vi "Serial Channel IO.vi"(0 "arm":bool, 1 "reset":bool, 2 "common resources":T15={"sync pulse resources"={"sync pulse destination terminal"="", "sync100"="", "sync pulse source terminal"="", "imported sync pulse register"="", "generate sync pulse handshake"="", "enable sync pulse register"="", "sync pulse clock"=""}, "serial channel resources"={"sc 0"={"completed frames register"=""}, "sc 1"={"completed frames register"=""}, "sc 2"={"completed frames register"=""}, "sc 3"={"completed frames register"=""}, "sc 4"={"completed frames register"=""}, "sc 5"={"completed frames register"=""}, "sc 6"={"completed frames register"=""}, "sc 7"={"completed frames register"=""}}, "dram manager 0"={"DRAM class"=refnum, "process clock"="", "registers"={"configuration"={"write time slice"="", "request time slice"="", "DRAM arbiter config"="", "partition config"=""}, "reset"={"handshake"={"start.go"="", "start.go rcvd"="", "done.go"="", "done.go rcvd"=""}, "process"={"in"="", "out"=""}, "write"={"in"="", "out 0"="", "out 1"="", "out 2"="", "out 3"=""}, "read"={"in"="", "out 0"="", "out 1"="", "out 2"="", "out 3"=""}}, "status"={"partition full"=""}}, "FIFOs"={"write data"={"FIFO 0"="", "FIFO 1"="", "FIFO 2"="", "FIFO 3"=""}, "request metadata"={"FIFO"=""}, "read data VOQ"={"FIFO 0"="", "FIFO 1"="", "FIFO 2"="", "FIFO 3"=""}, "read data"={"FIFO 0"="", "FIFO 1"="", "FIFO 2"="", "FIFO 3"=""}}, "num active streams"=0.0, "max open read requests"=256}, "dram manager 1"={"DRAM class"=refnum, "process clock"="", "registers"={"configuration"={"write time slice"="", "request time slice"="", "DRAM arbiter config"="", "partition config"=""}, "reset"={"handshake"={"start.go"="", "start.go rcvd"="", "done.go"="", "done.go rcvd"=""}, "process"={"in"="", "out"=""}, "write"={"in"="", "out 0"="", "out 1"="", "out 2"="", "out 3"=""}, "read"={"in"="", "out 0"="", "out 1"="", "out 2"="", "out 3"=""}}, "status"={"partition full"=""}}, "FIFOs"={"write data"={"FIFO 0"="", "FIFO 1"="", "FIFO 2"="", "FIFO 3"=""}, "request metadata"={"FIFO"=""}, "read data VOQ"={"FIFO 0"="", "FIFO 1"="", "FIFO 2"="", "FIFO 3"=""}, "read data"={"FIFO 0"="", "FIFO 1"="", "FIFO 2"="", "FIFO 3"=""}}, "num active streams"=0.0, "max open read requests"=256}}, 5 "stop":bool, 7 "timestamp counter value":T26, 9 "channel configs":T11[](array[typedef]) {"channel acq config"."first packet data type select mask" format="%.0x"; "channel acq config"."last packet data type select mask" format="%.0x"}, 11 "dram partition configs":T14[](array[typedef])=[{"first address"=0, "last address"=0}, {"first address"=0, "last address"=0}, {"first address"=0, "last address"=0}, {"first address"=0, "last address"=0}, {"first address"=0, "last address"=0}, {"first address"=0, "last address"=0}, {"first address"=0, "last address"=0}, {"first address"=0, "last address"=0}], 12 "ready for output":bool[](array[boolean])=[TRUE, TRUE, TRUE, TRUE, TRUE, TRUE, TRUE, TRUE]) -> (3 "acquisition error":bool, 4 "tagged llp packets cluster":T1, 6 "end of data":bool[](array[boolean]), 8 "serial input channel status":T27[](array[typedef])=[{"acq state"=enum."Idle", "stop timed out"=FALSE, "bad packet header"=FALSE, "bad packet payload"=FALSE, "bad packet size"=FALSE, "dram status"={"bytes written"=0, "bytes read"=0, "overflow"=FALSE, "partition full"=FALSE, "last byte flushed"=FALSE}}, {"acq state"=enum."Idle", "stop timed out"=FALSE, "bad packet header"=FALSE, "bad packet payload"=FALSE, "bad packet size"=FALSE, "dram status"={"bytes written"=0, "bytes read"=0, "overflow"=FALSE, "partition full"=FALSE, "last byte flushed"=FALSE}}, {"acq state"=enum."Idle", "stop timed out"=FALSE, "bad packet header"=FALSE, "bad packet payload"=FALSE, "bad packet size"=FALSE, "dram status"={"bytes written"=0, "bytes read"=0, "overflow"=FALSE, "partition full"=FALSE, "last byte flushed"=FALSE}}, {"acq state"=enum."Idle", "stop timed out"=FALSE, "bad packet header"=FALSE, "bad packet payload"=FALSE, "bad packet size"=FALSE, "dram status"={"bytes written"=0, "bytes read"=0, "overflow"=FALSE, "partition full"=FALSE, "last byte flushed"=FALSE}}, {"acq state"=enum."Idle", "stop timed out"=FALSE, "bad packet header"=FALSE, "bad packet payload"=FALSE, "bad packet size"=FALSE, "dram status"={"bytes written"=0, "bytes read"=0, "overflow"=FALSE, "partition full"=FALSE, "last byte flushed"=FALSE}}, {"acq state"=enum."Idle", "stop timed out"=FALSE, "bad packet header"=FALSE, "bad packet payload"=FALSE, "bad packet size"=FALSE, "dram status"={"bytes written"=0, "bytes read"=0, "overflow"=FALSE, "partition full"=FALSE, "last byte flushed"=FALSE}}, {"acq state"=enum."Idle", "stop timed out"=FALSE, "bad packet header"=FALSE, "bad packet payload"=FALSE, "bad packet size"=FALSE, "dram status"={"bytes written"=0, "bytes read"=0, "overflow"=FALSE, "partition full"=FALSE, "last byte flushed"=FALSE}}, {"acq state"=enum."Idle", "stop timed out"=FALSE, "bad packet header"=FALSE, "bad packet payload"=FALSE, "bad packet size"=FALSE, "dram status"={"bytes written"=0, "bytes read"=0, "overflow"=FALSE, "partition full"=FALSE, "last byte flushed"=FALSE}}], 10 "tagged llp packet valid":bool[](array[boolean]), 14 "ready for arm":bool, 15 "i2c monitor array":T13[](array[typedef]) {"monitor word" format="%.0x"})   [LabVIEW 2020, in "GettingStarted_Acq_Tap_148X_FPGA.lvlib"]
uses:
  GettingStarted_Acq_Tap_148X_FPGA.lvlib
  Types/Serial Input Channel Status.ctl
  <instrlib>/FlexRIO/CSI-2/v2/FPGA/Types/Channel-Based Acquisition Engine State.ctl
  Common/Types/DRAM Status.ctl
  <instrlib>/FlexRIO/CSI-2/v2/FPGA/Types/Timestamp Counter Value.ctl
  Common/Types/Common Resources.ctl
  <instrlib>/_niInstr/Memory/v1/FPGA/DRAM/niInstr Memory DRAM v1 FPGA.lvclass
  <instrlib>/FlexRIO/CSI-2/v2/FPGA/Types/Sync Pulse Resources.ctl
  Common/Types/Serial Channel Resources.ctl
  Common/Types/Single Serial Channel Resources.ctl
  <instrlib>/FlexRIO/CSI-2/v2/FPGA/DRAM Manager/Private/DRAM Manager.ctl
  <instrlib>/FlexRIO/CSI-2/v2/FPGA/DRAM Manager/Private/Common/DRAM Manager Registers.ctl
  <instrlib>/FlexRIO/CSI-2/v2/FPGA/DRAM Manager/Private/Common/Handshake Registers.ctl
  <instrlib>/FlexRIO/CSI-2/v2/FPGA/DRAM Manager/Private/Common/DRAM Manager FIFOs.ctl
  <instrlib>/FlexRIO/CSI-2/v2/FPGA/DRAM Manager/Private/Common/Write Data FIFO Ref.ctl
  <instrlib>/FlexRIO/CSI-2/v2/FPGA/DRAM Manager/Private/Common/Read Request Metadata FIFO Ref.ctl
  <instrlib>/FlexRIO/CSI-2/v2/FPGA/DRAM Manager/Private/Common/Read Data FIFO Ref.ctl
  <instrlib>/FlexRIO/CSI-2/v2/FPGA/DRAM Manager/Public/Partition Range.ctl
  <instrlib>/FlexRIO/API/FPGA/v1/IO/NI148x/i2c monitor.ctl
  Types/Serial Input Channel Datapath Configuration.ctl
  <instrlib>/FlexRIO/CSI-2/v2/FPGA/Types/Channel-Based Acquistion Engine Configuration.ctl
  Common/Types/Tagged LLP Packets Cluster.ctl
  <instrlib>/FlexRIO/CSI-2/v2/FPGA/Types/Tagged LLP Packet.ctl
  <instrlib>/FlexRIO/CSI-2/v2/FPGA/Types/FPGA LLP Packet Tag.ctl
  <instrlib>/FlexRIO/CSI-2/v2/FPGA/Types/FPGA LLP Packet Timestamp.ctl
  <instrlib>/FlexRIO/CSI-2/v2/FPGA/Types/Timestamp ID.ctl
  <instrlib>/FlexRIO/CSI-2/v2/FPGA/Types/FPGA LLP Packet Size.ctl
  <instrlib>/FlexRIO/CSI-2/v2/FPGA/Types/LLP Packet.ctl
  <instrlib>/FlexRIO/CSI-2/v2/FPGA/Types/LLP Packet Header.ctl
  <instrlib>/FlexRIO/CSI-2/v2/FPGA/Types/LLP Packet Payload.ctl
  <instrlib>/FlexRIO/CSI-2/v2/FPGA/Types/LLP Packet Footer.ctl
  <instrlib>/_niInstr/Basic Elements/v1/FPGA/niInstr Basic Elements v1 FPGA.lvlib
  Common/GettingStarted_Common_148X_FPGA.lvlib
  <instrlib>/FlexRIO/CSI-2/v2/FPGA/NI CSI-2 API FPGA v2.lvlib
  <instrlib>/FlexRIO/CSI-2/v2/FPGA/DRAM Manager/DRAM Manager v2.lvlib
  <instrlib>/FlexRIO/API/FPGA/v1/IO/NI148x/FlexRIO 148x FPGA v1.lvlib
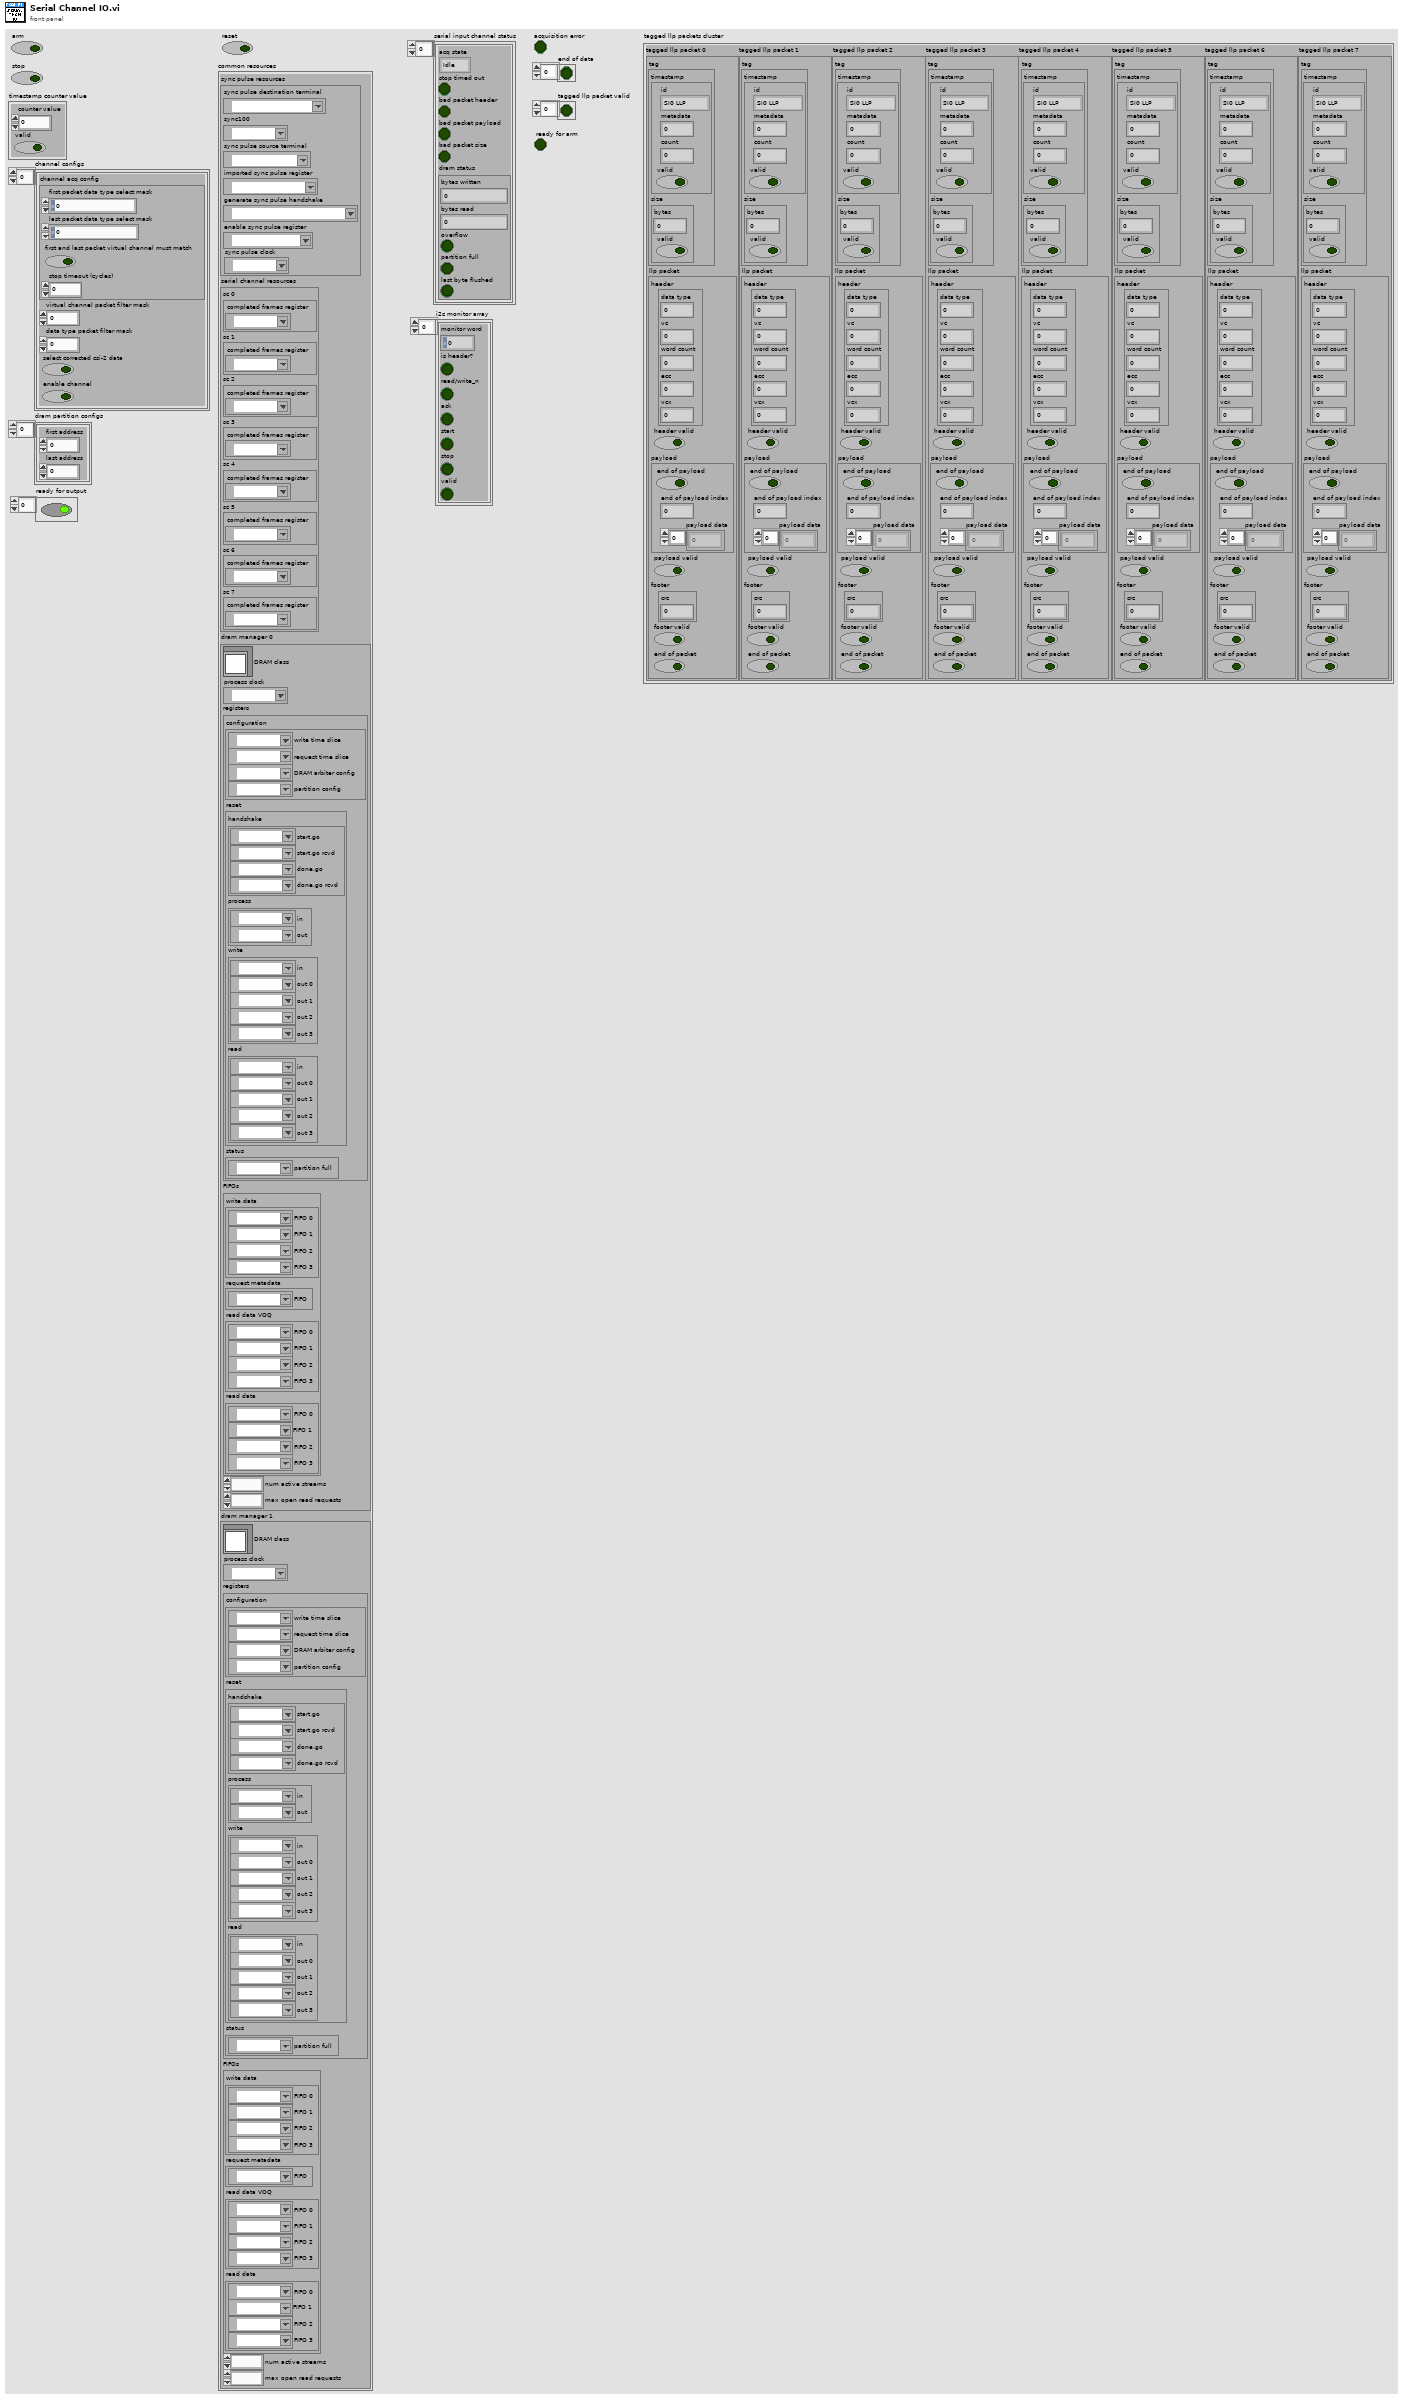
[diagram p1: front panel]
types:
  T1 = typedef "GettingStarted_Common_148X_FPGA.lvlib/Tagged LLP Packets Cluster.ctl" = cluster{"tagged llp packet 0":T2, "tagged llp packet 1":T2, "tagged llp packet 2":T2, "tagged llp packet 3":T2, "tagged llp packet 4":T2, "tagged llp packet 5":T2, "tagged llp packet 6":T2, "tagged llp packet 7":T2}
  T2 = typedef "NI CSI-2 API FPGA v2.lvlib/Tagged LLP Packet.ctl" = cluster{"tag":T3, "llp packet":T7}
  T3 = typedef "NI CSI-2 API FPGA v2.lvlib/FPGA LLP Packet Tag.ctl" = cluster{"timestamp":T4, "size":T6}
  T4 = typedef "NI CSI-2 API FPGA v2.lvlib/FPGA LLP Packet Timestamp.ctl" = cluster{"valid":bool, "count":fxp<+,50,50>, "id":T5, "metadata":u8}
  T5 = typedef "NI CSI-2 API FPGA v2.lvlib/Timestamp ID.ctl" = enum8{"SI0 LLP", "SI1 LLP", "SI2 LLP", "SI3 LLP", "SI4 LLP", "SI5 LLP", "SI6 LLP", "SI7 LLP", "SO0 LLP", "SO1 LLP", "SO2 LLP", "SO3 LLP", "SO4 LLP", "SO5 LLP", "SO6 LLP", "SO7 LLP", "Ser0 GPIO Bank", "Ser1 GPIO Bank", "Ser2 GPIO Bank", "Ser3 GPIO Bank", "Ser4 GPIO Bank", "Ser5 GPIO Bank", "Ser6 GPIO Bank", "Ser7 GPIO Bank", "Des0 GPIO Bank", "Des1 GPIO Bank", "Des2 GPIO Bank", "Des3 GPIO Bank", "Des4 GPIO Bank", "Des5 GPIO Bank", "Des6 GPIO Bank", "Des7 GPIO Bank", "User0", "User1", "User2", "User3", "User4", "User5", "User6", "User7", "User8", "User9", "User10", "User11", "User12", "User13", "User14", "User15", "User16", "User17", "User18", "User19", "User20", "User21", "User22", "User23", "User24", "User25", "User26", "User27", "User28", "User29", "User30", "User31"}
  T6 = typedef "NI CSI-2 API FPGA v2.lvlib/FPGA LLP Packet Size.ctl" = cluster{"bytes":fxp<+,17,17>, "valid":bool}
  T7 = typedef "NI CSI-2 API FPGA v2.lvlib/LLP Packet.ctl" = cluster{"header":T8, "header valid":bool, "payload":T9, "payload valid":bool, "footer":T10, "footer valid":bool, "end of packet":bool}
  T8 = typedef "NI CSI-2 API FPGA v2.lvlib/LLP Packet Header.ctl" = cluster{"word count":u16, "ecc":fxp<+,6,6>, "vcx":fxp<+,2,2>, "data type":fxp<+,6,6>, "vc":fxp<+,2,2>}
  T9 = typedef "NI CSI-2 API FPGA v2.lvlib/LLP Packet Payload.ctl" = cluster{"end of payload":bool, "end of payload index":fxp<+,3,3>, "payload data":u8[]}
  T10 = typedef "NI CSI-2 API FPGA v2.lvlib/LLP Packet Footer.ctl" = cluster{"crc":u16}
  T11 = typedef "GettingStarted_Acq_Tap_148X_FPGA.lvlib/Serial Input Channel Datapath Configuration.ctl" = cluster{"channel acq config":T12, "virtual channel packet filter mask":u16, "data type packet filter mask":u64, "select corrected csi-2 data":bool, "enable channel":bool}
  T12 = typedef "NI CSI-2 API FPGA v2.lvlib/Channel-Based Acquistion Engine Configuration.ctl" = cluster{"stop timeout (cycles)":u32, "first packet data type select mask":u64, "last packet data type select mask":u64, "first and last packet virtual channel must match":bool}
  T13 = typedef "FlexRIO 148x FPGA v1.lvlib/i2c monitor.ctl" = cluster{"monitor word":u8, "is header?":bool, "read/write_n":bool, "ack":bool, "start":bool, "stop":bool, "valid":bool}
  T14 = typedef "DRAM Manager v2.lvlib/Partition Range.ctl" = cluster{"first address":u32, "last address":u32}
  T15 = typedef "GettingStarted_Common_148X_FPGA.lvlib/Common Resources.ctl" = cluster{"sync pulse resources":T16, "serial channel resources":T17, "dram manager 0":T19, "dram manager 1":T19}
  T16 = typedef "NI CSI-2 API FPGA v2.lvlib/Sync Pulse Resources.ctl" = cluster{"sync pulse destination terminal":refnum<k21>, "sync100":refnum<k21>, "sync pulse source terminal":refnum<k21>, "imported sync pulse register":refnum<k21>, "generate sync pulse handshake":refnum<k21>, "enable sync pulse register":refnum<k21>, "sync pulse clock":refnum<k21>}
  T17 = typedef "GettingStarted_Common_148X_FPGA.lvlib/Serial Channel Resources.ctl" = cluster{"sc 0":T18, "sc 1":T18, "sc 2":T18, "sc 3":T18, "sc 4":T18, "sc 5":T18, "sc 6":T18, "sc 7":T18}
  T18 = typedef "GettingStarted_Common_148X_FPGA.lvlib/Single Serial Channel Resources.ctl" = cluster{"completed frames register":refnum<k21>}
  T19 = typedef "DRAM Manager v2.lvlib/DRAM Manager.ctl" = cluster{"DRAM class":refnum<class "niInstr Memory DRAM v1 FPGA.lvclass">, "process clock":refnum<k21>, "registers":T20, "FIFOs":T22, "num active streams":fxp<+,3,3>, "max open read requests":u16}
  T20 = typedef "DRAM Manager v2.lvlib/DRAM Manager Registers.ctl" = cluster{"configuration":cluster{"write time slice":refnum<k21>, "request time slice":refnum<k21>, "DRAM arbiter config":refnum<k21>, "partition config":refnum<k21>}, "reset":cluster{"handshake":T21, "process":cluster{"in":refnum<k21>, "out":refnum<k21>}, "write":cluster{"in":refnum<k21>, "out 0":refnum<k21>, "out 1":refnum<k21>, "out 2":refnum<k21>, "out 3":refnum<k21>}, "read":cluster{"in":refnum<k21>, "out 0":refnum<k21>, "out 1":refnum<k21>, "out 2":refnum<k21>, "out 3":refnum<k21>}}, "status":cluster{"partition full":refnum<k21>}}
  T21 = typedef "DRAM Manager v2.lvlib/Handshake Registers.ctl" = cluster{"start.go":refnum<k21>, "start.go rcvd":refnum<k21>, "done.go":refnum<k21>, "done.go rcvd":refnum<k21>}
  T22 = typedef "DRAM Manager v2.lvlib/DRAM Manager FIFOs.ctl" = cluster{"write data":cluster{"FIFO 0":T23, "FIFO 1":T23, "FIFO 2":T23, "FIFO 3":T23}, "request metadata":cluster{"FIFO":T24}, "read data VOQ":cluster{"FIFO 0":T25, "FIFO 1":T25, "FIFO 2":T25, "FIFO 3":T25}, "read data":cluster{"FIFO 0":T25, "FIFO 1":T25, "FIFO 2":T25, "FIFO 3":T25}}
  T23 = typedef "DRAM Manager v2.lvlib/Write Data FIFO Ref.ctl" = refnum<k21>
  T24 = typedef "DRAM Manager v2.lvlib/Read Request Metadata FIFO Ref.ctl" = refnum<k21>
  T25 = typedef "DRAM Manager v2.lvlib/Read Data FIFO Ref.ctl" = refnum<k21>
  T26 = typedef "NI CSI-2 API FPGA v2.lvlib/Timestamp Counter Value.ctl" = cluster{"counter value":u64, "valid":bool}
  T27 = typedef "GettingStarted_Acq_Tap_148X_FPGA.lvlib/Serial Input Channel Status.ctl" = cluster{"acq state":T28, "stop timed out":bool, "bad packet header":bool, "bad packet payload":bool, "bad packet size":bool, "dram status":T29}
  T28 = typedef "NI CSI-2 API FPGA v2.lvlib/Channel-Based Acquisition Engine State.ctl" = enum8{"Idle", "Wait for First Packet Header", "Acquire", "Wait for Last Packet Header", "Wait for End of Last Packet"}
  T29 = typedef "GettingStarted_Common_148X_FPGA.lvlib/DRAM Status.ctl" = cluster{"bytes written":u64, "bytes read":u64, "overflow":bool, "partition full":bool, "last byte flushed":bool}
  T30 = typedef "GettingStarted_Acq_Tap_148X_FPGA.lvlib/8 In Channel Resources.ctl" = cluster{"si 0 resources":T31, "si 1 resources":T31, "si 2 resources":T31, "si 3 resources":T31, "si 4 resources":T31, "si 5 resources":T31, "si 6 resources":T31, "si 7 resources":T31}
  T31 = typedef "GettingStarted_Acq_Tap_148X_FPGA.lvlib/Serial Input Channel Resources.ctl" = cluster{"dram manager":T19, "csi-2 input io":T32, "serial input channel instance":u8, "dram stream id":fxp<+,2,2>, "i2c io":T35}
  T32 = typedef "GettingStarted_Acq_Tap_148X_FPGA.lvlib/Serial Input Channel IO.ctl" = cluster{"32b":T33, "64b":T34, "csi-2 axi stream tlast":refnum<k21>, "csi-2 axi stream tvalid":refnum<k21>}
  T33 = typedef "GettingStarted_Acq_Tap_148X_FPGA.lvlib/Serial Input Channel IO 32b.ctl" = cluster{"csi-2 axi stream tdata":refnum<k21>, "csi-2 axi stream raw tdata":refnum<k21>, "csi-2 axi stream tuser":refnum<k21>}
  T34 = typedef "GettingStarted_Acq_Tap_148X_FPGA.lvlib/Serial Input Channel IO 64b.ctl" = cluster{"csi-2 axi stream tdata":refnum<k21>, "csi-2 axi stream raw tdata":refnum<k21>, "csi-2 axi stream tuser":refnum<k21>}
  T35 = typedef "GettingStarted_Common_148X_FPGA.lvlib/I2C IO.ctl" = cluster{"sda input":refnum<k21>, "sda output enable":refnum<k21>, "scl input":refnum<k21>, "scl output enable":refnum<k21>}
  T36 = cluster{"end of data":bool, "channel status":T27, "tagged llp packet valid":bool}
  T37 = cluster{"end of data":bool, "channel status":T27, "tagged llp packet valid":bool}[]
  T38 = typedef "GettingStarted_Acq_Tap_148X_FPGA.lvlib/4 In Channel Resources.ctl" = cluster{"si 0 resources":T31, "si 1 resources":T31, "si 2 resources":T31, "si 3 resources":T31}
  T39 = typedef "GettingStarted_Acq_Tap_148X_FPGA.lvlib/4 In 4 Out Channel Resources.ctl" = cluster{"si 0 resources":T31, "si 1 resources":T31, "si 2 resources":T31, "si 3 resources":T31, "so 0 resources":T40, "so 1 resources":T40, "so 2 resources":T40, "so 3 resources":T40}
  T40 = typedef "GettingStarted_Acq_Tap_148X_FPGA.lvlib/Serial Ouput Channel Resources.ctl" = cluster{"csi-2 output io":T41, "i2c io":T35}
  T41 = typedef "GettingStarted_Common_148X_FPGA.lvlib/Serial Output Channel IO.ctl" = cluster{"32b":T42, "64b":T43, "csi-2 axi stream tready":refnum<k21>, "csi-2 axi stream tvalid":refnum<k21>, "csi-2 axi stream tlast":refnum<k21>, "num packets in tx fifo":refnum<k21>, "ready to transmit packet":refnum<k21>, "transmit packet done":refnum<k21>, "transmit packet":refnum<k21>}
  T42 = typedef "GettingStarted_Common_148X_FPGA.lvlib/Serial Output Channel IO 32b.ctl" = cluster{"csi-2 axi stream tdata":refnum<k21>, "csi-2 axi stream tuser":refnum<k21>}
  T43 = typedef "GettingStarted_Common_148X_FPGA.lvlib/Serial Output Channel IO 64b.ctl" = cluster{"csi-2 axi stream tdata":refnum<k21>, "csi-2 axi stream tuser":refnum<k21>}
  T44 = typedef "GettingStarted_Acq_Tap_148X_FPGA.lvlib/2 In 2 Out Channel Resources.ctl" = cluster{"si 0 resources":T31, "si 1 resources":T31, "so 0 resources":T40, "so 1 resources":T40}
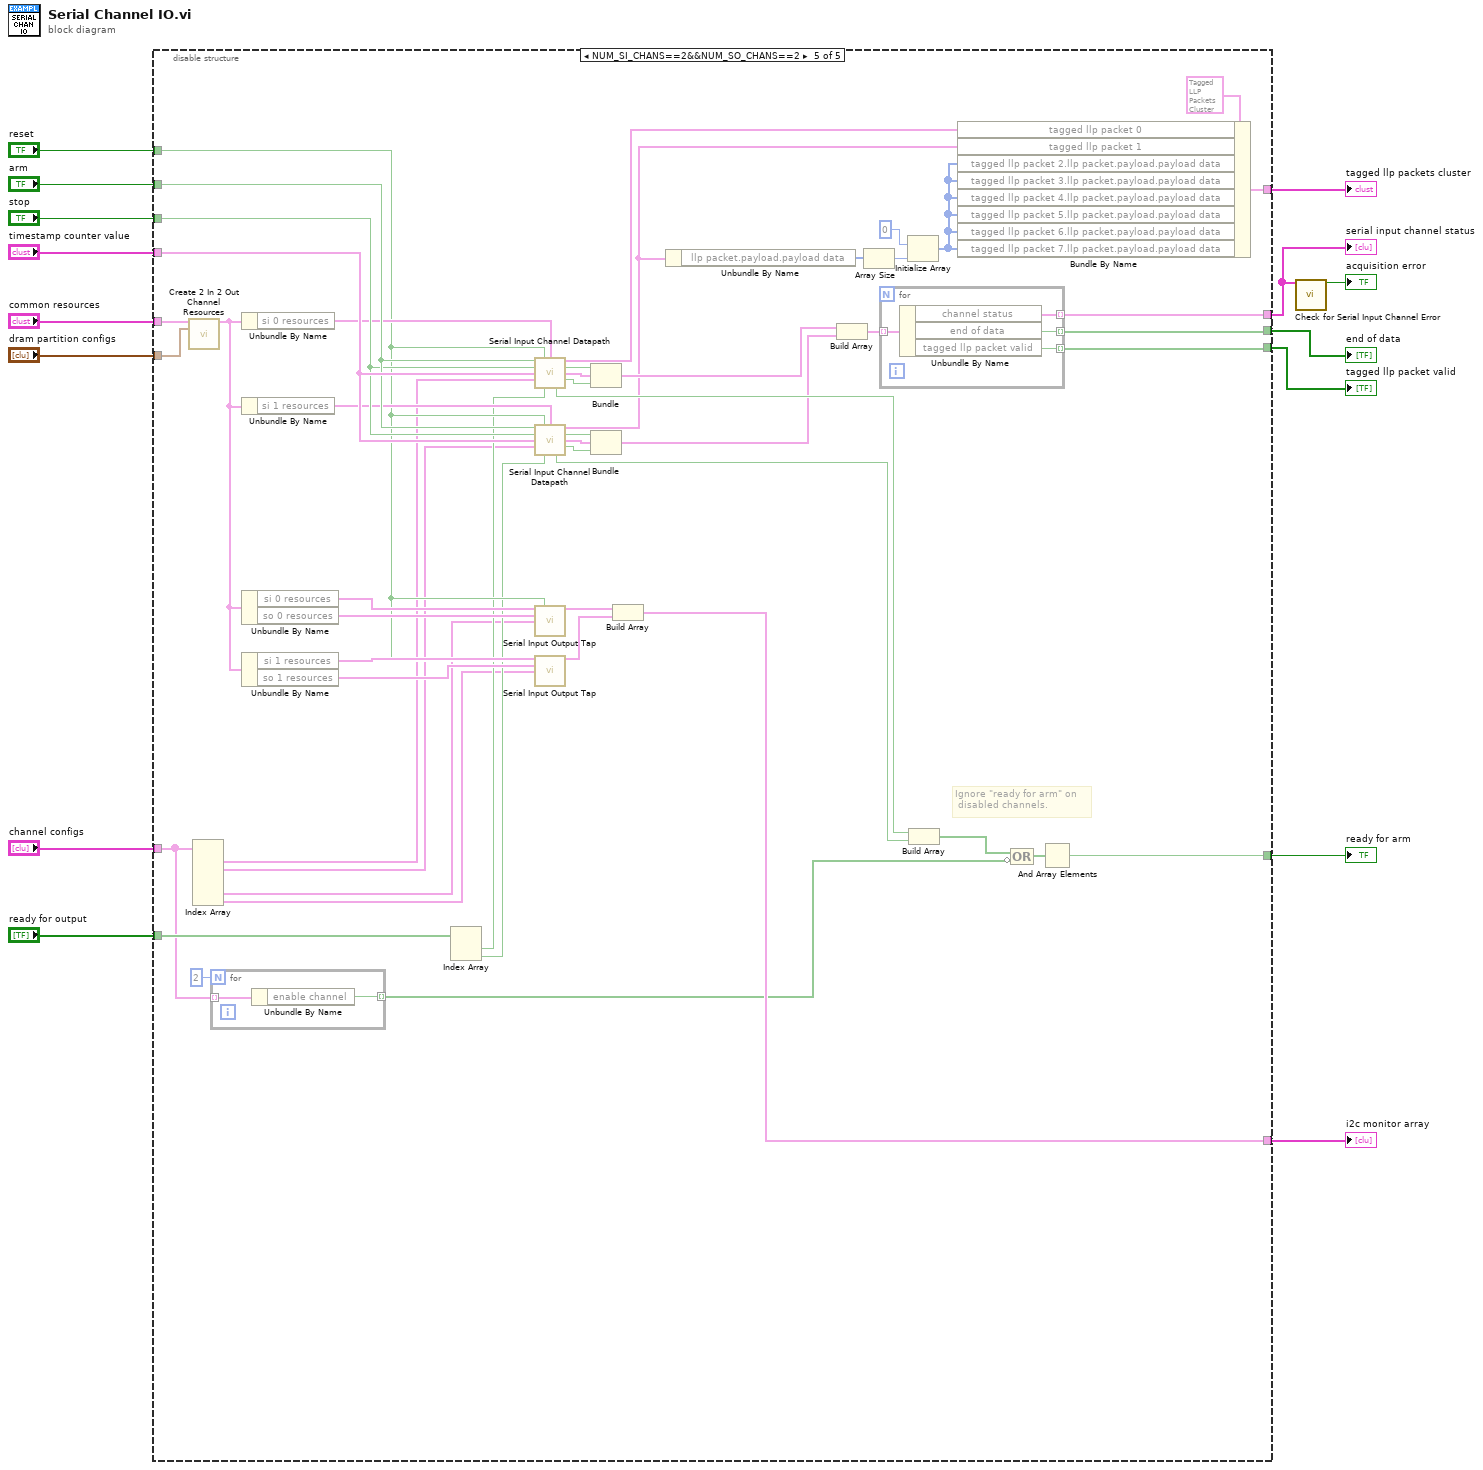
[diagram p0: block diagram]
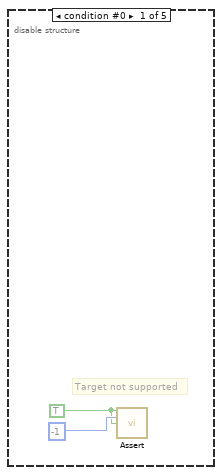
[diagram p2: hidden frame]
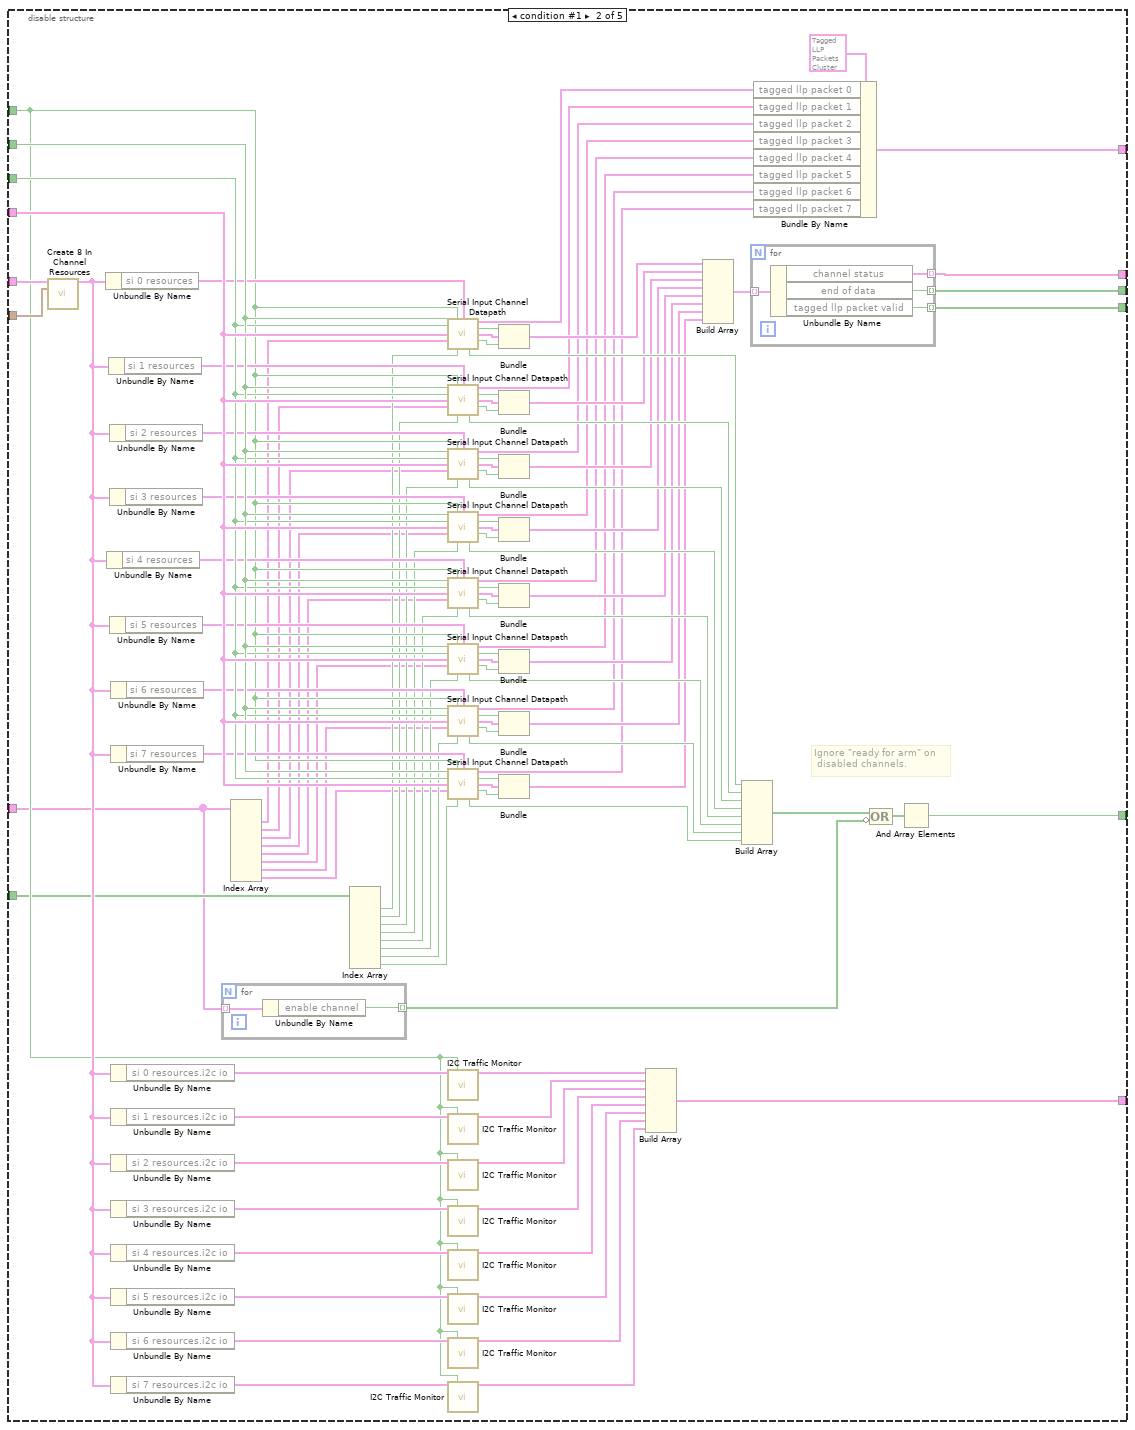
[diagram p3: hidden frame]
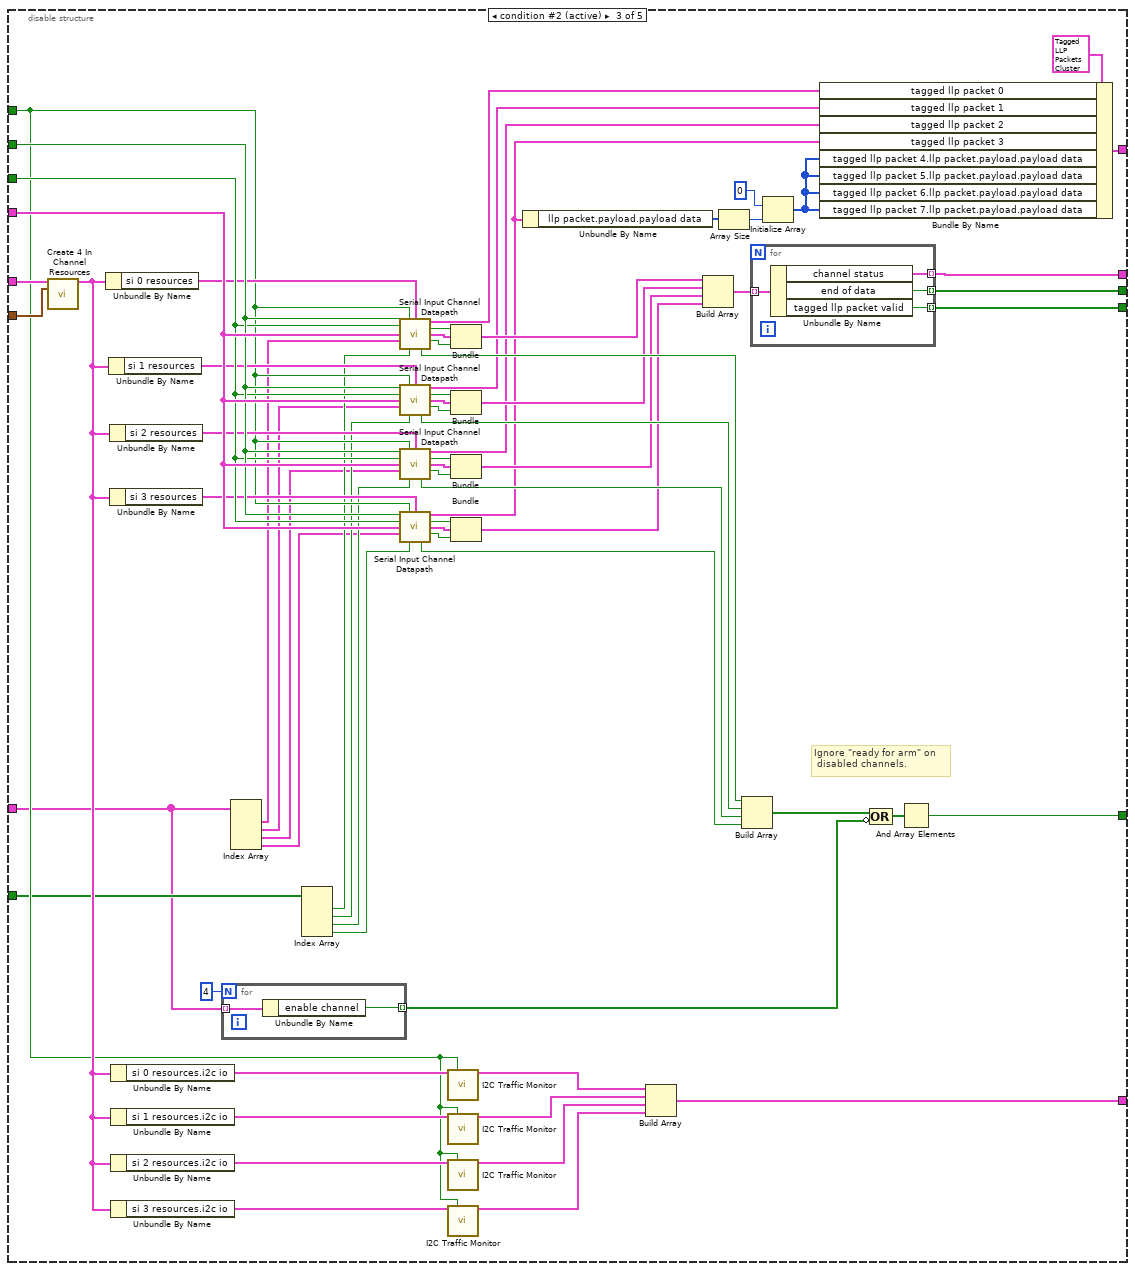
[diagram p4: hidden frame]
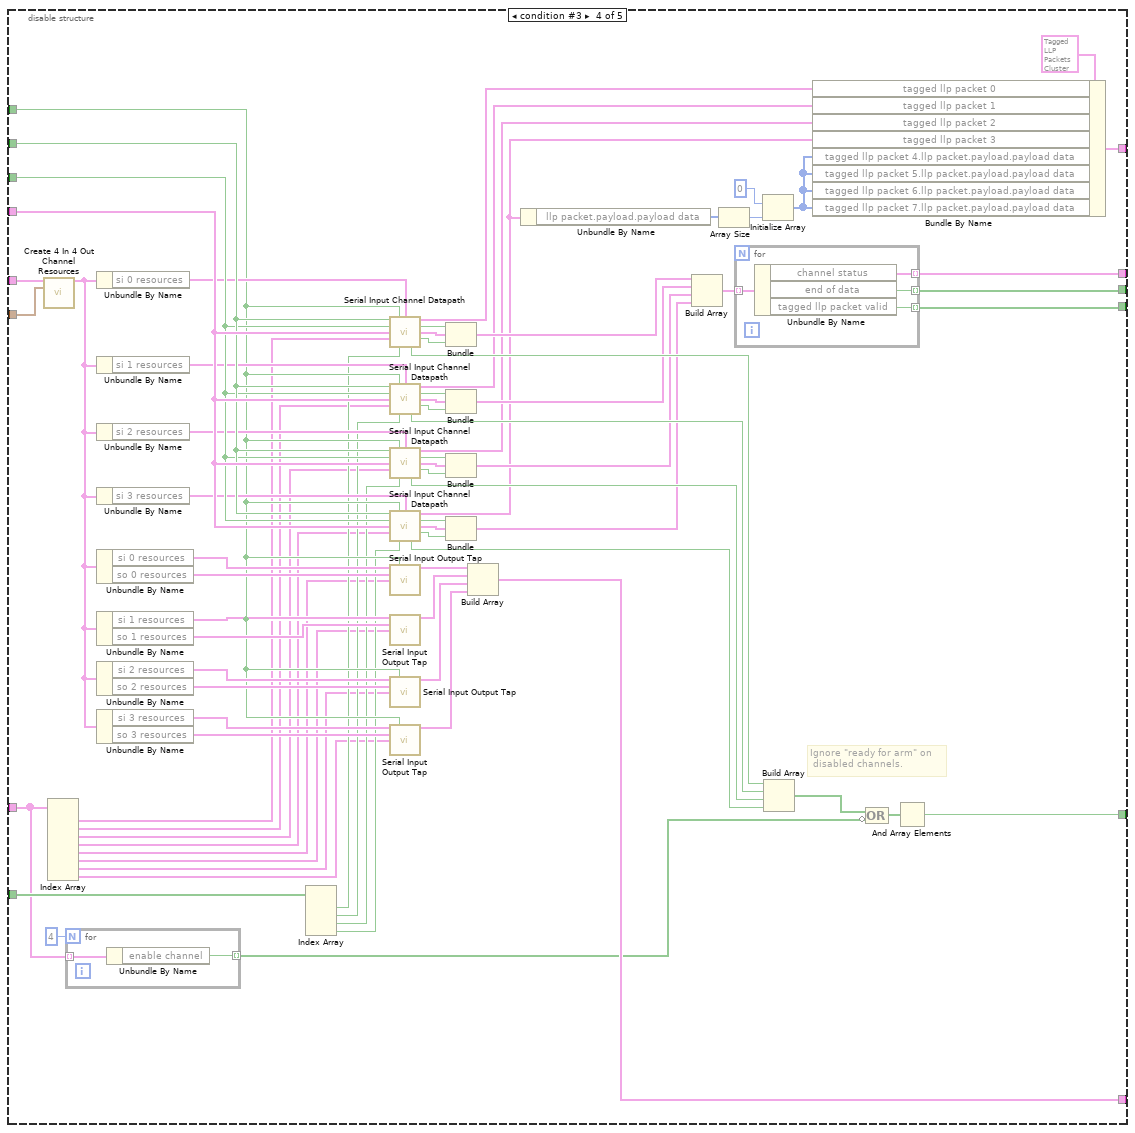
[diagram p5: hidden frame]
diagram:
  n1 = disable-structure shown="NUM_SI_CHANS==2&&NUM_SO_CHANS==2" {
    disable-tunnel: [_ w40 w151 w235 w310] -> w8
    disable-tunnel: "dram partition configs" -> [_ w103 w186 w258 w323]
    disable-tunnel: "timestamp counter value" -> [_ w125 w200 w283 w340]
    disable-tunnel: "reset" -> [_ w83 w174 w260 w325]
    disable-tunnel: "arm" -> [_ w120 w199 w282 w339]
    disable-tunnel: "stop" -> [_ w119 w198 w281 w338]
    disable-tunnel: "channel configs" -> [_ w36 w147 w219 w300]
    disable-tunnel: "common resources" -> [_ w102 w185 w259 w324]
    disable-tunnel: [_ w105 w188 w270 w331] -> w9
    disable-tunnel: [_ w99 w182 w253 w320] -> w6
    disable-tunnel: "ready for output" -> [_ w82 w173 w232 w307]
    disable-tunnel: [_ w39 w150 w233 w308] -> w4
    disable-tunnel: [_ w38 w149 w234 w309] -> w3
    disable-tunnel: [_ w26 w141 w215 w296] -> w1
    frame condition #0 {
      w16 = TRUE ("assert")
      # "Target not supported"
      n2 = call <instrlib>:"Assert.vi"("assert"=w16, "error code"=-1, "enable show error"=w16) -> ()  [unwired: 13 in]
    }
    frame condition #1 {
      # "Ignore \"ready for arm\" on\n disabled channels."
      n3 = call "Create 8 In Channel Resources.vi"("common resources"=w102, "dram partition configs"=w103) -> ("channel resources"=w91:T30)  [unwired: 13 in]
      n4 = Unbundle By Name(w91) -> ("si 0 resources"=w112:T31)
      n5 = Unbundle By Name(w91) -> ("si 4 resources"=w107:T31)
      n6 = Unbundle By Name(w91) -> ("si 1 resources"=w113:T31)
      n7 = Unbundle By Name(w91) -> ("si 2 resources"=w116:T31)
      n8 = Unbundle By Name(w91) -> ("si 3 resources"=w115:T31)
      n9 = Unbundle By Name(w91) -> ("si 5 resources"=w108:T31)
      n10 = Unbundle By Name(w91) -> ("si 6 resources"=w110:T31)
      n11 = Unbundle By Name(w91) -> ("si 7 resources"=w109:T31)
      n12 = Unbundle By Name(w91) -> ("si 0 resources.i2c io"=w101:T35)
      n13 = Unbundle By Name(w91) -> ("si 1 resources.i2c io"=w98:T35)
      n14 = Unbundle By Name(w91) -> ("si 2 resources.i2c io"=w97:T35)
      n15 = Unbundle By Name(w91) -> ("si 3 resources.i2c io"=w96:T35)
      n16 = Unbundle By Name(w91) -> ("si 4 resources.i2c io"=w95:T35)
      n17 = Unbundle By Name(w91) -> ("si 5 resources.i2c io"=w94:T35)
      n18 = Unbundle By Name(w91) -> ("si 6 resources.i2c io"=w93:T35)
      n19 = Unbundle By Name(w91) -> ("si 7 resources.i2c io"=w92:T35)
      n20 = for {
        tunnel: w36 -> [w127] mode=indexing
        tunnel: [w126] -> w37 mode=indexing
        n21 = Unbundle By Name(w127) -> ("enable channel"=w126:bool)
      }
      n22 = Index Array(array=w36) -> (element #1=w35:T11, element #2=w28:T11, element #3=w29:T11, element #4=w30:T11, element #5=w31:T11, element #6=w32:T11, element #7=w33:T11, element #8=w34:T11)  [unwired: 8 in]
      n23 = Index Array(array=w82) -> (element #1=w81:bool, element #2=w80:bool, element #3=w79:bool, element #4=w78:bool, element #5=w77:bool, element #6=w76:bool, element #7=w75:bool, element #8=w74:bool)  [unwired: 8 in]
      n24 = call "Serial Input Channel Datapath.vi"("arm"=w120, "reset"=w83, "resources"=w112, "stop"=w119, "timestamp counter value"=w125, "configuration"=w35, "ready for output"=w81) -> ("tagged llp packet"=w18:T2, "end of data"=w72:bool, "channel status"=w71:T27, "tagged llp packet valid"=w70:bool, "ready for arm"=w111:bool)  [unwired: 4 in]
      n25 = call "Serial Input Channel Datapath.vi"("arm"=w120, "reset"=w83, "resources"=w113, "stop"=w119, "timestamp counter value"=w125, "configuration"=w28, "ready for output"=w80) -> ("tagged llp packet"=w19:T2, "end of data"=w67:bool, "channel status"=w68:T27, "tagged llp packet valid"=w69:bool, "ready for arm"=w114:bool)  [unwired: 4 in]
      n26 = call "Serial Input Channel Datapath.vi"("arm"=w120, "reset"=w83, "resources"=w116, "stop"=w119, "timestamp counter value"=w125, "configuration"=w29, "ready for output"=w79) -> ("tagged llp packet"=w20:T2, "end of data"=w42:bool, "channel status"=w43:T27, "tagged llp packet valid"=w44:bool, "ready for arm"=w117:bool)  [unwired: 4 in]
      n27 = call "Serial Input Channel Datapath.vi"("arm"=w120, "reset"=w83, "resources"=w115, "stop"=w119, "timestamp counter value"=w125, "configuration"=w30, "ready for output"=w78) -> ("tagged llp packet"=w21:T2, "end of data"=w45:bool, "channel status"=w46:T27, "tagged llp packet valid"=w47:bool, "ready for arm"=w118:bool)  [unwired: 4 in]
      n28 = call "Serial Input Channel Datapath.vi"("arm"=w120, "reset"=w83, "resources"=w107, "stop"=w119, "timestamp counter value"=w125, "configuration"=w31, "ready for output"=w77) -> ("tagged llp packet"=w22:T2, "end of data"=w48:bool, "channel status"=w49:T27, "tagged llp packet valid"=w50:bool, "ready for arm"=w121:bool)  [unwired: 4 in]
      n29 = call "Serial Input Channel Datapath.vi"("arm"=w120, "reset"=w83, "resources"=w108, "stop"=w119, "timestamp counter value"=w125, "configuration"=w32, "ready for output"=w76) -> ("tagged llp packet"=w23:T2, "end of data"=w51:bool, "channel status"=w52:T27, "tagged llp packet valid"=w53:bool, "ready for arm"=w122:bool)  [unwired: 4 in]
      n30 = call "Serial Input Channel Datapath.vi"("arm"=w120, "reset"=w83, "resources"=w110, "stop"=w119, "timestamp counter value"=w125, "configuration"=w33, "ready for output"=w75) -> ("tagged llp packet"=w24:T2, "end of data"=w54:bool, "channel status"=w55:T27, "tagged llp packet valid"=w56:bool, "ready for arm"=w123:bool)  [unwired: 4 in]
      n31 = call "Serial Input Channel Datapath.vi"("arm"=w120, "reset"=w83, "resources"=w109, "stop"=w119, "timestamp counter value"=w125, "configuration"=w34, "ready for output"=w74) -> ("tagged llp packet"=w25:T2, "end of data"=w57:bool, "channel status"=w58:T27, "tagged llp packet valid"=w59:bool, "ready for arm"=w124:bool)  [unwired: 4 in]
      n32 = call "I2C Traffic Monitor.vi"("channel i2c io"=w101, "reset"=w83) -> ("i2c monitor"=w100:T13)  [unwired: 13 in]
      n33 = call "I2C Traffic Monitor.vi"("channel i2c io"=w98, "reset"=w83) -> ("i2c monitor"=w90:T13)  [unwired: 13 in]
      n34 = call "I2C Traffic Monitor.vi"("channel i2c io"=w97, "reset"=w83) -> ("i2c monitor"=w89:T13)  [unwired: 13 in]
      n35 = call "I2C Traffic Monitor.vi"("channel i2c io"=w96, "reset"=w83) -> ("i2c monitor"=w88:T13)  [unwired: 13 in]
      n36 = call "I2C Traffic Monitor.vi"("channel i2c io"=w95, "reset"=w83) -> ("i2c monitor"=w87:T13)  [unwired: 13 in]
      n37 = call "I2C Traffic Monitor.vi"("channel i2c io"=w94, "reset"=w83) -> ("i2c monitor"=w86:T13)  [unwired: 13 in]
      n38 = call "I2C Traffic Monitor.vi"("channel i2c io"=w93, "reset"=w83) -> ("i2c monitor"=w85:T13)  [unwired: 13 in]
      n39 = call "I2C Traffic Monitor.vi"("channel i2c io"=w92, "reset"=w83) -> ("i2c monitor"=w84:T13)  [unwired: 13 in]
      n40 = Bundle("end of data"=w72, "channel status"=w71, "tagged llp packet valid"=w70) -> (w73:T36)  [unwired: 1 in]
      n41 = Bundle("end of data"=w67, "channel status"=w68, "tagged llp packet valid"=w69) -> (w66:T36)  [unwired: 1 in]
      n42 = Bundle("end of data"=w42, "channel status"=w43, "tagged llp packet valid"=w44) -> (w60:T36)  [unwired: 1 in]
      n43 = Bundle("end of data"=w45, "channel status"=w46, "tagged llp packet valid"=w47) -> (w61:T36)  [unwired: 1 in]
      n44 = Bundle("end of data"=w48, "channel status"=w49, "tagged llp packet valid"=w50) -> (w62:T36)  [unwired: 1 in]
      n45 = Bundle("end of data"=w51, "channel status"=w52, "tagged llp packet valid"=w53) -> (w63:T36)  [unwired: 1 in]
      n46 = Bundle("end of data"=w54, "channel status"=w55, "tagged llp packet valid"=w56) -> (w64:T36)  [unwired: 1 in]
      n47 = Bundle("end of data"=w57, "channel status"=w58, "tagged llp packet valid"=w59) -> (w65:T36)  [unwired: 1 in]
      n48 = Build Array(w100, w90, w89, w88, w87, w86, w85, w84) -> (w99:T13[])
      n49 = Build Array(w73, w66, w60, w61, w62, w63, w64, w65) -> (w41:T37)
      n50 = Build Array(w111, w114, w117, w118, w121, w122, w123, w124) -> (w104:bool[])
      n51 = for {
        tunnel: w41 -> [w131] mode=indexing
        tunnel: [w130] -> w40 mode=indexing
        tunnel: [w129] -> w39 mode=indexing
        tunnel: [w128] -> w38 mode=indexing
        n52 = Unbundle By Name(w131) -> ("channel status"=w130:T27, "end of data"=w128:bool, "tagged llp packet valid"=w129:bool)
      }
      n53 = Bundle By Name(cluster=T1 {"tagged llp packet 0"={"tag"={"timestamp"={"valid"=FALSE, "count"=0.0, "id"=enum."SI0 LLP", "metadata"=0}, "size"={"bytes"=0.0, "valid"=FALSE}}, "llp packet"={"header"={"word count"=0, "ecc"=0.0, "vcx"=0.0, "data type"=0.0, "vc"=0.0}, "header valid"=FALSE, "payload"={"end of payload"=FALSE, "end of payload index"=0.0, "payload data"=[0, 0, 0, 0]}, "payload valid"=FALSE, "footer"={"crc"=0}, "footer valid"=FALSE, "end of packet"=FALSE}}, "tagged llp packet 1"={"tag"={"timestamp"={"valid"=FALSE, "count"=0.0, "id"=enum."SI0 LLP", "metadata"=0}, "size"={"bytes"=0.0, "valid"=FALSE}}, "llp packet"={"header"={"word count"=0, "ecc"=0.0, "vcx"=0.0, "data type"=0.0, "vc"=0.0}, "header valid"=FALSE, "payload"={"end of payload"=FALSE, "end of payload index"=0.0, "payload data"=[0, 0, 0, 0]}, "payload valid"=FALSE, "footer"={"crc"=0}, "footer valid"=FALSE, "end of packet"=FALSE}}, "tagged llp packet 2"={"tag"={"timestamp"={"valid"=FALSE, "count"=0.0, "id"=enum."SI0 LLP", "metadata"=0}, "size"={"bytes"=0.0, "valid"=FALSE}}, "llp packet"={"header"={"word count"=0, "ecc"=0.0, "vcx"=0.0, "data type"=0.0, "vc"=0.0}, "header valid"=FALSE, "payload"={"end of payload"=FALSE, "end of payload index"=0.0, "payload data"=[0, 0, 0, 0]}, "payload valid"=FALSE, "footer"={"crc"=0}, "footer valid"=FALSE, "end of packet"=FALSE}}, "tagged llp packet 3"={"tag"={"timestamp"={"valid"=FALSE, "count"=0.0, "id"=enum."SI0 LLP", "metadata"=0}, "size"={"bytes"=0.0, "valid"=FALSE}}, "llp packet"={"header"={"word count"=0, "ecc"=0.0, "vcx"=0.0, "data type"=0.0, "vc"=0.0}, "header valid"=FALSE, "payload"={"end of payload"=FALSE, "end of payload index"=0.0, "payload data"=[0, 0, 0, 0]}, "payload valid"=FALSE, "footer"={"crc"=0}, "footer valid"=FALSE, "end of packet"=FALSE}}, "tagged llp packet 4"={"tag"={"timestamp"={"valid"=FALSE, "count"=0.0, "id"=enum."SI0 LLP", "metadata"=0}, "size"={"bytes"=0.0, "valid"=FALSE}}, "llp packet"={"header"={"word count"=0, "ecc"=0.0, "vcx"=0.0, "data type"=0.0, "vc"=0.0}, "header valid"=FALSE, "payload"={"end of payload"=FALSE, "end of payload index"=0.0, "payload data"=[0, 0, 0, 0]}, "payload valid"=FALSE, "footer"={"crc"=0}, "footer valid"=FALSE, "end of packet"=FALSE}}, "tagged llp packet 5"={"tag"={"timestamp"={"valid"=FALSE, "count"=0.0, "id"=enum."SI0 LLP", "metadata"=0}, "size"={"bytes"=0.0, "valid"=FALSE}}, "llp packet"={"header"={"word count"=0, "ecc"=0.0, "vcx"=0.0, "data type"=0.0, "vc"=0.0}, "header valid"=FALSE, "payload"={"end of payload"=FALSE, "end of payload index"=0.0, "payload data"=[0, 0, 0, 0]}, "payload valid"=FALSE, "footer"={"crc"=0}, "footer valid"=FALSE, "end of packet"=FALSE}}, "tagged llp packet 6"={"tag"={"timestamp"={"valid"=FALSE, "count"=0.0, "id"=enum."SI0 LLP", "metadata"=0}, "size"={"bytes"=0.0, "valid"=FALSE}}, "llp packet"={"header"={"word count"=0, "ecc"=0.0, "vcx"=0.0, "data type"=0.0, "vc"=0.0}, "header valid"=FALSE, "payload"={"end of payload"=FALSE, "end of payload index"=0.0, "payload data"=[0, 0, 0, 0]}, "payload valid"=FALSE, "footer"={"crc"=0}, "footer valid"=FALSE, "end of packet"=FALSE}}, "tagged llp packet 7"={"tag"={"timestamp"={"valid"=FALSE, "count"=0.0, "id"=enum."SI0 LLP", "metadata"=0}, "size"={"bytes"=0.0, "valid"=FALSE}}, "llp packet"={"header"={"word count"=0, "ecc"=0.0, "vcx"=0.0, "data type"=0.0, "vc"=0.0}, "header valid"=FALSE, "payload"={"end of payload"=FALSE, "end of payload index"=0.0, "payload data"=[0, 0, 0, 0]}, "payload valid"=FALSE, "footer"={"crc"=0}, "footer valid"=FALSE, "end of packet"=FALSE}}} ("tagged llp packets cluster out"), "tagged llp packet 0"=w18, "tagged llp packet 1"=w19, "tagged llp packet 2"=w20, "tagged llp packet 3"=w21, "tagged llp packet 4"=w22, "tagged llp packet 5"=w23, "tagged llp packet 6"=w24, "tagged llp packet 7"=w25) -> (w26:T1)
      n54 = Compound Arithmetic op=OR(w104, invert w37) -> (w106:bool[])
      n55 = And Array Elements(Boolean array=w106) -> (logical AND=w105:bool)
    }
    frame condition #2 (active) {
      # "Ignore \"ready for arm\" on\n disabled channels."
      n56 = call "Create 4 In Channel Resources.vi"("common resources"=w185, "dram partition configs"=w186) -> ("channel resources"=w178:T38)  [unwired: 13 in]
      n57 = Unbundle By Name(w178) -> ("si 0 resources"=w191:T31)
      n58 = Unbundle By Name(w178) -> ("si 1 resources"=w192:T31)
      n59 = Unbundle By Name(w178) -> ("si 2 resources"=w195:T31)
      n60 = Unbundle By Name(w178) -> ("si 3 resources"=w194:T31)
      n61 = Unbundle By Name(w178) -> ("si 0 resources.i2c io"=w184:T35)
      n62 = Unbundle By Name(w178) -> ("si 1 resources.i2c io"=w181:T35)
      n63 = Unbundle By Name(w178) -> ("si 2 resources.i2c io"=w180:T35)
      n64 = Unbundle By Name(w178) -> ("si 3 resources.i2c io"=w179:T35)
      n65 = for {
        N: 4 -> [_]
        tunnel: w147 -> [w202] mode=indexing
        tunnel: [w201] -> w148 mode=indexing
        n66 = Unbundle By Name(w202) -> ("enable channel"=w201:bool)
      }
      n67 = Index Array(array=w147) -> (element #1=w146:T11, element #2=w143:T11, element #3=w144:T11, element #4=w145:T11)  [unwired: 4 in]
      n68 = Index Array(array=w173) -> (element #1=w172:bool, element #2=w171:bool, element #3=w170:bool, element #4=w169:bool)  [unwired: 4 in]
      n69 = call "Serial Input Channel Datapath.vi"("arm"=w199, "reset"=w174, "resources"=w191, "stop"=w198, "timestamp counter value"=w200, "configuration"=w146, "ready for output"=w172) -> ("tagged llp packet"=w138:T2, "end of data"=w167:bool, "channel status"=w166:T27, "tagged llp packet valid"=w165:bool, "ready for arm"=w190:bool)  [unwired: 4 in]
      n70 = call "Serial Input Channel Datapath.vi"("arm"=w199, "reset"=w174, "resources"=w192, "stop"=w198, "timestamp counter value"=w200, "configuration"=w143, "ready for output"=w171) -> ("tagged llp packet"=w139:T2, "end of data"=w162:bool, "channel status"=w163:T27, "tagged llp packet valid"=w164:bool, "ready for arm"=w193:bool)  [unwired: 4 in]
      n71 = call "Serial Input Channel Datapath.vi"("arm"=w199, "reset"=w174, "resources"=w195, "stop"=w198, "timestamp counter value"=w200, "configuration"=w144, "ready for output"=w170) -> ("tagged llp packet"=w140:T2, "end of data"=w153:bool, "channel status"=w154:T27, "tagged llp packet valid"=w155:bool, "ready for arm"=w196:bool)  [unwired: 4 in]
      n72 = call "Serial Input Channel Datapath.vi"("arm"=w199, "reset"=w174, "resources"=w194, "stop"=w198, "timestamp counter value"=w200, "configuration"=w145, "ready for output"=w169) -> ("tagged llp packet"=w134:T2, "end of data"=w156:bool, "channel status"=w157:T27, "tagged llp packet valid"=w158:bool, "ready for arm"=w197:bool)  [unwired: 4 in]
      n73 = call "I2C Traffic Monitor.vi"("channel i2c io"=w184, "reset"=w174) -> ("i2c monitor"=w183:T13)  [unwired: 13 in]
      n74 = call "I2C Traffic Monitor.vi"("channel i2c io"=w181, "reset"=w174) -> ("i2c monitor"=w177:T13)  [unwired: 13 in]
      n75 = call "I2C Traffic Monitor.vi"("channel i2c io"=w180, "reset"=w174) -> ("i2c monitor"=w176:T13)  [unwired: 13 in]
      n76 = call "I2C Traffic Monitor.vi"("channel i2c io"=w179, "reset"=w174) -> ("i2c monitor"=w175:T13)  [unwired: 13 in]
      n77 = Bundle("end of data"=w167, "channel status"=w166, "tagged llp packet valid"=w165) -> (w168:T36)  [unwired: 1 in]
      n78 = Bundle("end of data"=w162, "channel status"=w163, "tagged llp packet valid"=w164) -> (w161:T36)  [unwired: 1 in]
      n79 = Bundle("end of data"=w153, "channel status"=w154, "tagged llp packet valid"=w155) -> (w159:T36)  [unwired: 1 in]
      n80 = Bundle("end of data"=w156, "channel status"=w157, "tagged llp packet valid"=w158) -> (w160:T36)  [unwired: 1 in]
      n81 = Unbundle By Name(w134) -> ("llp packet.payload.payload data"=w137:u8[])
      n82 = Build Array(w183, w177, w176, w175) -> (w182:T13[])
      n83 = Build Array(w168, w161, w159, w160) -> (w152:T37)
      n84 = Array Size(array=w137) -> (size(s)=w136:i32)
      n85 = Build Array(w190, w193, w196, w197) -> (w187:bool[])
      n86 = for {
        tunnel: w152 -> [w206] mode=indexing
        tunnel: [w205] -> w151 mode=indexing
        tunnel: [w204] -> w150 mode=indexing
        tunnel: [w203] -> w149 mode=indexing
        n87 = Unbundle By Name(w206) -> ("channel status"=w205:T27, "end of data"=w203:bool, "tagged llp packet valid"=w204:bool)
      }
      n88 = Initialize Array(u8 0 ("element"), w136) -> (w133:u8[])
      n89 = Bundle By Name(cluster=T1 {"tagged llp packet 0"={"tag"={"timestamp"={"valid"=FALSE, "count"=0.0, "id"=enum."SI0 LLP", "metadata"=0}, "size"={"bytes"=0.0, "valid"=FALSE}}, "llp packet"={"header"={"word count"=0, "ecc"=0.0, "vcx"=0.0, "data type"=0.0, "vc"=0.0}, "header valid"=FALSE, "payload"={"end of payload"=FALSE, "end of payload index"=0.0, "payload data"=[0, 0, 0, 0]}, "payload valid"=FALSE, "footer"={"crc"=0}, "footer valid"=FALSE, "end of packet"=FALSE}}, "tagged llp packet 1"={"tag"={"timestamp"={"valid"=FALSE, "count"=0.0, "id"=enum."SI0 LLP", "metadata"=0}, "size"={"bytes"=0.0, "valid"=FALSE}}, "llp packet"={"header"={"word count"=0, "ecc"=0.0, "vcx"=0.0, "data type"=0.0, "vc"=0.0}, "header valid"=FALSE, "payload"={"end of payload"=FALSE, "end of payload index"=0.0, "payload data"=[0, 0, 0, 0]}, "payload valid"=FALSE, "footer"={"crc"=0}, "footer valid"=FALSE, "end of packet"=FALSE}}, "tagged llp packet 2"={"tag"={"timestamp"={"valid"=FALSE, "count"=0.0, "id"=enum."SI0 LLP", "metadata"=0}, "size"={"bytes"=0.0, "valid"=FALSE}}, "llp packet"={"header"={"word count"=0, "ecc"=0.0, "vcx"=0.0, "data type"=0.0, "vc"=0.0}, "header valid"=FALSE, "payload"={"end of payload"=FALSE, "end of payload index"=0.0, "payload data"=[0, 0, 0, 0]}, "payload valid"=FALSE, "footer"={"crc"=0}, "footer valid"=FALSE, "end of packet"=FALSE}}, "tagged llp packet 3"={"tag"={"timestamp"={"valid"=FALSE, "count"=0.0, "id"=enum."SI0 LLP", "metadata"=0}, "size"={"bytes"=0.0, "valid"=FALSE}}, "llp packet"={"header"={"word count"=0, "ecc"=0.0, "vcx"=0.0, "data type"=0.0, "vc"=0.0}, "header valid"=FALSE, "payload"={"end of payload"=FALSE, "end of payload index"=0.0, "payload data"=[0, 0, 0, 0]}, "payload valid"=FALSE, "footer"={"crc"=0}, "footer valid"=FALSE, "end of packet"=FALSE}}, "tagged llp packet 4"={"tag"={"timestamp"={"valid"=FALSE, "count"=0.0, "id"=enum."SI0 LLP", "metadata"=0}, "size"={"bytes"=0.0, "valid"=FALSE}}, "llp packet"={"header"={"word count"=0, "ecc"=0.0, "vcx"=0.0, "data type"=0.0, "vc"=0.0}, "header valid"=FALSE, "payload"={"end of payload"=FALSE, "end of payload index"=0.0, "payload data"=[0, 0, 0, 0]}, "payload valid"=FALSE, "footer"={"crc"=0}, "footer valid"=FALSE, "end of packet"=FALSE}}, "tagged llp packet 5"={"tag"={"timestamp"={"valid"=FALSE, "count"=0.0, "id"=enum."SI0 LLP", "metadata"=0}, "size"={"bytes"=0.0, "valid"=FALSE}}, "llp packet"={"header"={"word count"=0, "ecc"=0.0, "vcx"=0.0, "data type"=0.0, "vc"=0.0}, "header valid"=FALSE, "payload"={"end of payload"=FALSE, "end of payload index"=0.0, "payload data"=[0, 0, 0, 0]}, "payload valid"=FALSE, "footer"={"crc"=0}, "footer valid"=FALSE, "end of packet"=FALSE}}, "tagged llp packet 6"={"tag"={"timestamp"={"valid"=FALSE, "count"=0.0, "id"=enum."SI0 LLP", "metadata"=0}, "size"={"bytes"=0.0, "valid"=FALSE}}, "llp packet"={"header"={"word count"=0, "ecc"=0.0, "vcx"=0.0, "data type"=0.0, "vc"=0.0}, "header valid"=FALSE, "payload"={"end of payload"=FALSE, "end of payload index"=0.0, "payload data"=[0, 0, 0, 0]}, "payload valid"=FALSE, "footer"={"crc"=0}, "footer valid"=FALSE, "end of packet"=FALSE}}, "tagged llp packet 7"={"tag"={"timestamp"={"valid"=FALSE, "count"=0.0, "id"=enum."SI0 LLP", "metadata"=0}, "size"={"bytes"=0.0, "valid"=FALSE}}, "llp packet"={"header"={"word count"=0, "ecc"=0.0, "vcx"=0.0, "data type"=0.0, "vc"=0.0}, "header valid"=FALSE, "payload"={"end of payload"=FALSE, "end of payload index"=0.0, "payload data"=[0, 0, 0, 0]}, "payload valid"=FALSE, "footer"={"crc"=0}, "footer valid"=FALSE, "end of packet"=FALSE}}} ("tagged llp packets cluster out"), "tagged llp packet 0"=w138, "tagged llp packet 1"=w139, "tagged llp packet 2"=w140, "tagged llp packet 3"=w134, "tagged llp packet 4.llp packet.payload.payload data"=w133, "tagged llp packet 5.llp packet.payload.payload data"=w133, "tagged llp packet 6.llp packet.payload.payload data"=w133, "tagged llp packet 7.llp packet.payload.payload data"=w133) -> (w141:T1)
      n90 = Compound Arithmetic op=OR(w187, invert w148) -> (w189:bool[])
      n91 = And Array Elements(Boolean array=w189) -> (logical AND=w188:bool)
    }
    frame condition #3 {
      # "Ignore \"ready for arm\" on\n disabled channels."
      n92 = call "Create 4 In 4 Out Channel Resources.vi"("common resources"=w259, "dram partition configs"=w258) -> ("channel resources"=w264:T39)  [unwired: 13 in]
      n93 = Index Array(array=w219) -> (element #1=w227:T11, element #2=w226:T11, element #3=w225:T11, element #4=w224:T11, element #5=w220:T11, element #6=w221:T11, element #7=w222:T11, element #8=w223:T11)  [unwired: 8 in]
      n94 = for {
        N: 4 -> [_]
        tunnel: w219 -> [w285] mode=indexing
        tunnel: [w284] -> w217 mode=indexing
        n95 = Unbundle By Name(w285) -> ("enable channel"=w284:bool)
      }
      n96 = Unbundle By Name(w264) -> ("si 0 resources"=w275:T31)
      n97 = Unbundle By Name(w264) -> ("si 1 resources"=w276:T31)
      n98 = Unbundle By Name(w264) -> ("si 2 resources"=w279:T31)
      n99 = Unbundle By Name(w264) -> ("si 3 resources"=w278:T31)
      n100 = Unbundle By Name(w264) -> ("si 0 resources"=w269:T31, "so 0 resources"=w268:T40)
      n101 = Unbundle By Name(w264) -> ("si 1 resources"=w261:T31, "so 1 resources"=w267:T40)
      n102 = Unbundle By Name(w264) -> ("si 2 resources"=w262:T31, "so 2 resources"=w266:T40)
      n103 = Unbundle By Name(w264) -> ("si 3 resources"=w263:T31, "so 3 resources"=w265:T40)
      n104 = Index Array(array=w232) -> (element #1=w228:bool, element #2=w229:bool, element #3=w230:bool, element #4=w231:bool)  [unwired: 4 in]
      n105 = call "Serial Input Channel Datapath.vi"("arm"=w282, "reset"=w260, "resources"=w275, "stop"=w281, "timestamp counter value"=w283, "configuration"=w227, "ready for output"=w228) -> ("tagged llp packet"=w212:T2, "end of data"=w249:bool, "channel status"=w250:T27, "tagged llp packet valid"=w252:bool, "ready for arm"=w274:bool)  [unwired: 4 in]
      n106 = call "Serial Input Channel Datapath.vi"("arm"=w282, "reset"=w260, "resources"=w276, "stop"=w281, "timestamp counter value"=w283, "configuration"=w226, "ready for output"=w229) -> ("tagged llp packet"=w213:T2, "end of data"=w237:bool, "channel status"=w238:T27, "tagged llp packet valid"=w239:bool, "ready for arm"=w277:bool)  [unwired: 4 in]
      n107 = call "Serial Input Channel Datapath.vi"("arm"=w282, "reset"=w260, "resources"=w279, "stop"=w281, "timestamp counter value"=w283, "configuration"=w225, "ready for output"=w230) -> ("tagged llp packet"=w214:T2, "end of data"=w240:bool, "channel status"=w241:T27, "tagged llp packet valid"=w242:bool, "ready for arm"=w280:bool)  [unwired: 4 in]
      n108 = call "Serial Input Channel Datapath.vi"("arm"=w282, "reset"=w260, "resources"=w278, "stop"=w281, "timestamp counter value"=w283, "configuration"=w224, "ready for output"=w231) -> ("tagged llp packet"=w211:T2, "end of data"=w243:bool, "channel status"=w244:T27, "tagged llp packet valid"=w245:bool, "ready for arm"=w273:bool)  [unwired: 4 in]
      n109 = call "Serial Input Output Tap.vi"("serial input channel resources"=w269, "reset"=w260, "serial output channel resources"=w268, "datapath config"=w220) -> ("i2c monitor"=w257:T13)  [unwired: 11 in]
      n110 = call "Serial Input Output Tap.vi"("serial input channel resources"=w261, "reset"=w260, "serial output channel resources"=w267, "datapath config"=w221) -> ("i2c monitor"=w256:T13)  [unwired: 11 in]
      n111 = call "Serial Input Output Tap.vi"("serial input channel resources"=w262, "reset"=w260, "serial output channel resources"=w266, "datapath config"=w222) -> ("i2c monitor"=w255:T13)  [unwired: 11 in]
      n112 = call "Serial Input Output Tap.vi"("serial input channel resources"=w263, "reset"=w260, "serial output channel resources"=w265, "datapath config"=w223) -> ("i2c monitor"=w254:T13)  [unwired: 11 in]
      n113 = Bundle("end of data"=w249, "channel status"=w250, "tagged llp packet valid"=w252) -> (w251:T36)  [unwired: 1 in]
      n114 = Bundle("end of data"=w237, "channel status"=w238, "tagged llp packet valid"=w239) -> (w248:T36)  [unwired: 1 in]
      n115 = Bundle("end of data"=w240, "channel status"=w241, "tagged llp packet valid"=w242) -> (w247:T36)  [unwired: 1 in]
      n116 = Bundle("end of data"=w243, "channel status"=w244, "tagged llp packet valid"=w245) -> (w246:T36)  [unwired: 1 in]
      n117 = Build Array(w257, w256, w255, w254) -> (w253:T13[])
      n118 = Unbundle By Name(w211) -> ("llp packet.payload.payload data"=w210:u8[])
      n119 = Build Array(w251, w248, w247, w246) -> (w236:T37)
      n120 = Array Size(array=w210) -> (size(s)=w209:i32)
      n121 = for {
        tunnel: w236 -> [w289] mode=indexing
        tunnel: [w288] -> w235 mode=indexing
        tunnel: [w287] -> w233 mode=indexing
        tunnel: [w286] -> w234 mode=indexing
        n122 = Unbundle By Name(w289) -> ("channel status"=w288:T27, "end of data"=w286:bool, "tagged llp packet valid"=w287:bool)
      }
      n123 = Initialize Array(u8 0 ("element"), w209) -> (w207:u8[])
      n124 = Build Array(w274, w277, w280, w273) -> (w271:bool[])
      n125 = Bundle By Name(cluster=T1 {"tagged llp packet 0"={"tag"={"timestamp"={"valid"=FALSE, "count"=0.0, "id"=enum."SI0 LLP", "metadata"=0}, "size"={"bytes"=0.0, "valid"=FALSE}}, "llp packet"={"header"={"word count"=0, "ecc"=0.0, "vcx"=0.0, "data type"=0.0, "vc"=0.0}, "header valid"=FALSE, "payload"={"end of payload"=FALSE, "end of payload index"=0.0, "payload data"=[0, 0, 0, 0]}, "payload valid"=FALSE, "footer"={"crc"=0}, "footer valid"=FALSE, "end of packet"=FALSE}}, "tagged llp packet 1"={"tag"={"timestamp"={"valid"=FALSE, "count"=0.0, "id"=enum."SI0 LLP", "metadata"=0}, "size"={"bytes"=0.0, "valid"=FALSE}}, "llp packet"={"header"={"word count"=0, "ecc"=0.0, "vcx"=0.0, "data type"=0.0, "vc"=0.0}, "header valid"=FALSE, "payload"={"end of payload"=FALSE, "end of payload index"=0.0, "payload data"=[0, 0, 0, 0]}, "payload valid"=FALSE, "footer"={"crc"=0}, "footer valid"=FALSE, "end of packet"=FALSE}}, "tagged llp packet 2"={"tag"={"timestamp"={"valid"=FALSE, "count"=0.0, "id"=enum."SI0 LLP", "metadata"=0}, "size"={"bytes"=0.0, "valid"=FALSE}}, "llp packet"={"header"={"word count"=0, "ecc"=0.0, "vcx"=0.0, "data type"=0.0, "vc"=0.0}, "header valid"=FALSE, "payload"={"end of payload"=FALSE, "end of payload index"=0.0, "payload data"=[0, 0, 0, 0]}, "payload valid"=FALSE, "footer"={"crc"=0}, "footer valid"=FALSE, "end of packet"=FALSE}}, "tagged llp packet 3"={"tag"={"timestamp"={"valid"=FALSE, "count"=0.0, "id"=enum."SI0 LLP", "metadata"=0}, "size"={"bytes"=0.0, "valid"=FALSE}}, "llp packet"={"header"={"word count"=0, "ecc"=0.0, "vcx"=0.0, "data type"=0.0, "vc"=0.0}, "header valid"=FALSE, "payload"={"end of payload"=FALSE, "end of payload index"=0.0, "payload data"=[0, 0, 0, 0]}, "payload valid"=FALSE, "footer"={"crc"=0}, "footer valid"=FALSE, "end of packet"=FALSE}}, "tagged llp packet 4"={"tag"={"timestamp"={"valid"=FALSE, "count"=0.0, "id"=enum."SI0 LLP", "metadata"=0}, "size"={"bytes"=0.0, "valid"=FALSE}}, "llp packet"={"header"={"word count"=0, "ecc"=0.0, "vcx"=0.0, "data type"=0.0, "vc"=0.0}, "header valid"=FALSE, "payload"={"end of payload"=FALSE, "end of payload index"=0.0, "payload data"=[0, 0, 0, 0]}, "payload valid"=FALSE, "footer"={"crc"=0}, "footer valid"=FALSE, "end of packet"=FALSE}}, "tagged llp packet 5"={"tag"={"timestamp"={"valid"=FALSE, "count"=0.0, "id"=enum."SI0 LLP", "metadata"=0}, "size"={"bytes"=0.0, "valid"=FALSE}}, "llp packet"={"header"={"word count"=0, "ecc"=0.0, "vcx"=0.0, "data type"=0.0, "vc"=0.0}, "header valid"=FALSE, "payload"={"end of payload"=FALSE, "end of payload index"=0.0, "payload data"=[0, 0, 0, 0]}, "payload valid"=FALSE, "footer"={"crc"=0}, "footer valid"=FALSE, "end of packet"=FALSE}}, "tagged llp packet 6"={"tag"={"timestamp"={"valid"=FALSE, "count"=0.0, "id"=enum."SI0 LLP", "metadata"=0}, "size"={"bytes"=0.0, "valid"=FALSE}}, "llp packet"={"header"={"word count"=0, "ecc"=0.0, "vcx"=0.0, "data type"=0.0, "vc"=0.0}, "header valid"=FALSE, "payload"={"end of payload"=FALSE, "end of payload index"=0.0, "payload data"=[0, 0, 0, 0]}, "payload valid"=FALSE, "footer"={"crc"=0}, "footer valid"=FALSE, "end of packet"=FALSE}}, "tagged llp packet 7"={"tag"={"timestamp"={"valid"=FALSE, "count"=0.0, "id"=enum."SI0 LLP", "metadata"=0}, "size"={"bytes"=0.0, "valid"=FALSE}}, "llp packet"={"header"={"word count"=0, "ecc"=0.0, "vcx"=0.0, "data type"=0.0, "vc"=0.0}, "header valid"=FALSE, "payload"={"end of payload"=FALSE, "end of payload index"=0.0, "payload data"=[0, 0, 0, 0]}, "payload valid"=FALSE, "footer"={"crc"=0}, "footer valid"=FALSE, "end of packet"=FALSE}}} ("tagged llp packets cluster out"), "tagged llp packet 0"=w212, "tagged llp packet 1"=w213, "tagged llp packet 2"=w214, "tagged llp packet 3"=w211, "tagged llp packet 4.llp packet.payload.payload data"=w207, "tagged llp packet 5.llp packet.payload.payload data"=w207, "tagged llp packet 6.llp packet.payload.payload data"=w207, "tagged llp packet 7.llp packet.payload.payload data"=w207) -> (w215:T1)
      n126 = Compound Arithmetic op=OR(w271, invert w217) -> (w272:bool[])
      n127 = And Array Elements(Boolean array=w272) -> (logical AND=w270:bool)
    }
    frame condition #4 {
      # "Ignore \"ready for arm\" on\n disabled channels."
      n128 = call "Create 2 In 2 Out Channel Resources.vi"("common resources"=w324, "dram partition configs"=w323) -> ("channel resources"=w327:T44)  [unwired: 13 in]
      n129 = Index Array(array=w300) -> (element #1=w304:T11, element #2=w303:T11, element #5=w301:T11, element #6=w302:T11)  [unwired: 6 in, 2 out]
      n130 = for {
        N: 2 -> [_]
        tunnel: w300 -> [w342] mode=indexing
        tunnel: [w341] -> w298 mode=indexing
        n131 = Unbundle By Name(w342) -> ("enable channel"=w341:bool)
      }
      n132 = Unbundle By Name(w327) -> ("si 0 resources"=w335:T31)
      n133 = Unbundle By Name(w327) -> ("si 1 resources"=w336:T31)
      n134 = Unbundle By Name(w327) -> ("si 0 resources"=w330:T31, "so 0 resources"=w329:T40)
      n135 = Unbundle By Name(w327) -> ("si 1 resources"=w326:T31, "so 1 resources"=w328:T40)
      n136 = Index Array(array=w307) -> (element #1=w305:bool, element #2=w306:bool)  [unwired: 2 in]
      n137 = call "Serial Input Channel Datapath.vi"("arm"=w339, "reset"=w325, "resources"=w335, "stop"=w338, "timestamp counter value"=w340, "configuration"=w304, "ready for output"=w305) -> ("tagged llp packet"=w295:T2, "end of data"=w316:bool, "channel status"=w317:T27, "tagged llp packet valid"=w319:bool, "ready for arm"=w334:bool)  [unwired: 4 in]
      n138 = call "Serial Input Channel Datapath.vi"("arm"=w339, "reset"=w325, "resources"=w336, "stop"=w338, "timestamp counter value"=w340, "configuration"=w303, "ready for output"=w306) -> ("tagged llp packet"=w291:T2, "end of data"=w312:bool, "channel status"=w313:T27, "tagged llp packet valid"=w314:bool, "ready for arm"=w337:bool)  [unwired: 4 in]
      n139 = call "Serial Input Output Tap.vi"("serial input channel resources"=w330, "reset"=w325, "serial output channel resources"=w329, "datapath config"=w301) -> ("i2c monitor"=w322:T13)  [unwired: 11 in]
      n140 = call "Serial Input Output Tap.vi"("serial input channel resources"=w326, "reset"=w325, "serial output channel resources"=w328, "datapath config"=w302) -> ("i2c monitor"=w321:T13)  [unwired: 11 in]
      n141 = Bundle("end of data"=w316, "channel status"=w317, "tagged llp packet valid"=w319) -> (w318:T36)  [unwired: 1 in]
      n142 = Bundle("end of data"=w312, "channel status"=w313, "tagged llp packet valid"=w314) -> (w315:T36)  [unwired: 1 in]
      n143 = Build Array(w322, w321) -> (w320:T13[])
      n144 = Unbundle By Name(w291) -> ("llp packet.payload.payload data"=w294:u8[])
      n145 = Build Array(w318, w315) -> (w311:T37)
      n146 = Array Size(array=w294) -> (size(s)=w293:i32)
      n147 = for {
        tunnel: w311 -> [w346] mode=indexing
        tunnel: [w345] -> w310 mode=indexing
        tunnel: [w344] -> w308 mode=indexing
        tunnel: [w343] -> w309 mode=indexing
        n148 = Unbundle By Name(w346) -> ("channel status"=w345:T27, "end of data"=w343:bool, "tagged llp packet valid"=w344:bool)
      }
      n149 = Initialize Array(u8 0 ("element"), w293) -> (w290:u8[])
      n150 = Build Array(w334, w337) -> (w332:bool[])
      n151 = Bundle By Name(cluster=T1 {"tagged llp packet 0"={"tag"={"timestamp"={"valid"=FALSE, "count"=0.0, "id"=enum."SI0 LLP", "metadata"=0}, "size"={"bytes"=0.0, "valid"=FALSE}}, "llp packet"={"header"={"word count"=0, "ecc"=0.0, "vcx"=0.0, "data type"=0.0, "vc"=0.0}, "header valid"=FALSE, "payload"={"end of payload"=FALSE, "end of payload index"=0.0, "payload data"=[0, 0, 0, 0]}, "payload valid"=FALSE, "footer"={"crc"=0}, "footer valid"=FALSE, "end of packet"=FALSE}}, "tagged llp packet 1"={"tag"={"timestamp"={"valid"=FALSE, "count"=0.0, "id"=enum."SI0 LLP", "metadata"=0}, "size"={"bytes"=0.0, "valid"=FALSE}}, "llp packet"={"header"={"word count"=0, "ecc"=0.0, "vcx"=0.0, "data type"=0.0, "vc"=0.0}, "header valid"=FALSE, "payload"={"end of payload"=FALSE, "end of payload index"=0.0, "payload data"=[0, 0, 0, 0]}, "payload valid"=FALSE, "footer"={"crc"=0}, "footer valid"=FALSE, "end of packet"=FALSE}}, "tagged llp packet 2"={"tag"={"timestamp"={"valid"=FALSE, "count"=0.0, "id"=enum."SI0 LLP", "metadata"=0}, "size"={"bytes"=0.0, "valid"=FALSE}}, "llp packet"={"header"={"word count"=0, "ecc"=0.0, "vcx"=0.0, "data type"=0.0, "vc"=0.0}, "header valid"=FALSE, "payload"={"end of payload"=FALSE, "end of payload index"=0.0, "payload data"=[0, 0, 0, 0]}, "payload valid"=FALSE, "footer"={"crc"=0}, "footer valid"=FALSE, "end of packet"=FALSE}}, "tagged llp packet 3"={"tag"={"timestamp"={"valid"=FALSE, "count"=0.0, "id"=enum."SI0 LLP", "metadata"=0}, "size"={"bytes"=0.0, "valid"=FALSE}}, "llp packet"={"header"={"word count"=0, "ecc"=0.0, "vcx"=0.0, "data type"=0.0, "vc"=0.0}, "header valid"=FALSE, "payload"={"end of payload"=FALSE, "end of payload index"=0.0, "payload data"=[0, 0, 0, 0]}, "payload valid"=FALSE, "footer"={"crc"=0}, "footer valid"=FALSE, "end of packet"=FALSE}}, "tagged llp packet 4"={"tag"={"timestamp"={"valid"=FALSE, "count"=0.0, "id"=enum."SI0 LLP", "metadata"=0}, "size"={"bytes"=0.0, "valid"=FALSE}}, "llp packet"={"header"={"word count"=0, "ecc"=0.0, "vcx"=0.0, "data type"=0.0, "vc"=0.0}, "header valid"=FALSE, "payload"={"end of payload"=FALSE, "end of payload index"=0.0, "payload data"=[0, 0, 0, 0]}, "payload valid"=FALSE, "footer"={"crc"=0}, "footer valid"=FALSE, "end of packet"=FALSE}}, "tagged llp packet 5"={"tag"={"timestamp"={"valid"=FALSE, "count"=0.0, "id"=enum."SI0 LLP", "metadata"=0}, "size"={"bytes"=0.0, "valid"=FALSE}}, "llp packet"={"header"={"word count"=0, "ecc"=0.0, "vcx"=0.0, "data type"=0.0, "vc"=0.0}, "header valid"=FALSE, "payload"={"end of payload"=FALSE, "end of payload index"=0.0, "payload data"=[0, 0, 0, 0]}, "payload valid"=FALSE, "footer"={"crc"=0}, "footer valid"=FALSE, "end of packet"=FALSE}}, "tagged llp packet 6"={"tag"={"timestamp"={"valid"=FALSE, "count"=0.0, "id"=enum."SI0 LLP", "metadata"=0}, "size"={"bytes"=0.0, "valid"=FALSE}}, "llp packet"={"header"={"word count"=0, "ecc"=0.0, "vcx"=0.0, "data type"=0.0, "vc"=0.0}, "header valid"=FALSE, "payload"={"end of payload"=FALSE, "end of payload index"=0.0, "payload data"=[0, 0, 0, 0]}, "payload valid"=FALSE, "footer"={"crc"=0}, "footer valid"=FALSE, "end of packet"=FALSE}}, "tagged llp packet 7"={"tag"={"timestamp"={"valid"=FALSE, "count"=0.0, "id"=enum."SI0 LLP", "metadata"=0}, "size"={"bytes"=0.0, "valid"=FALSE}}, "llp packet"={"header"={"word count"=0, "ecc"=0.0, "vcx"=0.0, "data type"=0.0, "vc"=0.0}, "header valid"=FALSE, "payload"={"end of payload"=FALSE, "end of payload index"=0.0, "payload data"=[0, 0, 0, 0]}, "payload valid"=FALSE, "footer"={"crc"=0}, "footer valid"=FALSE, "end of packet"=FALSE}}} ("tagged llp packets cluster out"), "tagged llp packet 0"=w295, "tagged llp packet 1"=w291, "tagged llp packet 2.llp packet.payload.payload data"=w290, "tagged llp packet 3.llp packet.payload.payload data"=w290, "tagged llp packet 4.llp packet.payload.payload data"=w290, "tagged llp packet 5.llp packet.payload.payload data"=w290, "tagged llp packet 6.llp packet.payload.payload data"=w290, "tagged llp packet 7.llp packet.payload.payload data"=w290) -> (w296:T1)
      n152 = Compound Arithmetic op=OR(w332, invert w298) -> (w333:bool[])
      n153 = And Array Elements(Boolean array=w333) -> (logical AND=w331:bool)
    }
  }
  "serial input channel status" <- w8
  "ready for arm" <- w9
  "i2c monitor array" <- w6
  "end of data" <- w3
  "tagged llp packet valid" <- w4
  "tagged llp packets cluster" <- w1
  n154 = call "Check for Serial Input Channel Error.vi"("serial input channel status"=w8) -> ("acquisition error"=→"acquisition error":bool)  [unwired: 14 in]
